vi "Get Thermocouple Meas Volt.vi"(8 "error in (no error)":errorcluster, 11 "VISA resource name":refnum<visa-resource-name>) -> (0 "error out":errorcluster, 2 "Meas Value":dbl format="%^.3e", 3 "VISA resource name out":refnum<visa-resource-name>)   [LabVIEW 2014, in "Fluke 5XXX Series Multicalibrators.lvlib"]
doc: "This VI returns the last value of the thermocouple temperature measurement in volts. If the last measurement was an overload or open thermocouple condition, or there is no measurement, returns 0E+00.\n\nNote:\n\nThis VI is available only for instrument models 5500A and 5520A."
uses:
  Fluke 5XXX Series Multicalibrators.lvlib
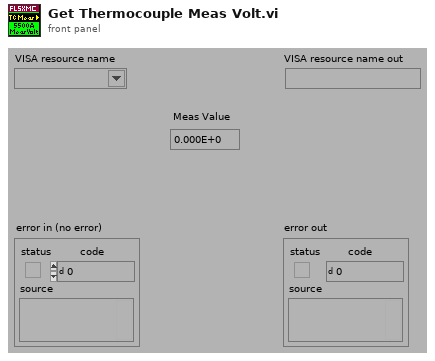
[diagram p1: front panel]
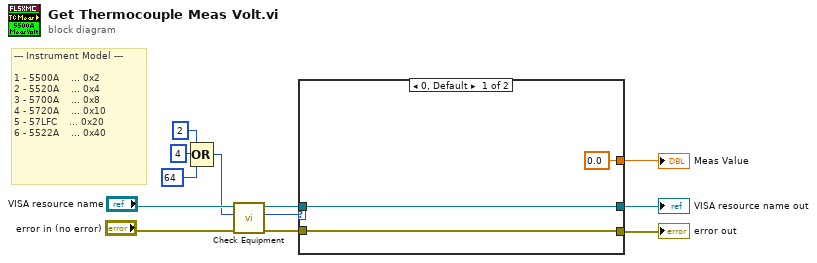
[diagram p0: block diagram]
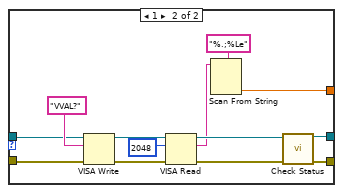
[diagram p2: hidden frame]
diagram:
  # "--- Instrument Model ---\n\n1 - 5500A    ... 0x2\n2 - 5520A    ... 0x4\n3 - 5700A    ... 0x8\n4 - 5720A    ... 0x10\n5 - 57LFC    ... 0x20\n6 - 5522A    ... 0x40"
  n1 = Compound Arithmetic op=OR(2 ("Numeric"), 4 ("Numeric"), 64 ("Numeric")) -> (w5:i32)
  n2 = call "Check Equipment.vi"("error in (no error)"="error in (no error)", "Bit Mask"=w5, "VISA resource name"="VISA resource name") -> ("error out"=w12:errorcluster, "Present?"=w10:u32, "VISA resource name out"=w11:refnum<visa-resource-name>)  [unwired: 6 in]
  n3 = case shown="0, Default" w10 {
    tunnel: [w15 w22] -> w3
    tunnel: [w14 w19] -> w2
    tunnel: w12 -> [w15 w24]
    tunnel: w11 -> [w14 w23]
    tunnel: [0.0 w16] -> w4
    frame 0, Default {
    }
    frame 1 {
      n4 = VISA Write(VISA resource name=w23, write buffer="VVAL?", error in (no error)=w24) -> (VISA resource name out=w27:refnum<visa-resource-name>, error out=w26:errorcluster)  [unwired: 1 out]
      n5 = VISA Read(VISA resource name=w27, byte count=u32 2048 ("byte count (0)"), error in (no error)=w26) -> (VISA resource name out=w20:refnum<visa-resource-name>, read buffer=w17:string, error out=w21:errorcluster)  [unwired: 1 out]
      n6 = Scan From String(format string="%.;%Le", input string=w17) -> (output 1=w16:dbl)  [unwired: 3 in, 3 out]
      n7 = call "Check Status.vi"("VISA resource name"=w20, "error in (no error)"=w21) -> ("VISA resource name out"=w19:refnum<visa-resource-name>, "error out"=w22:errorcluster)  [unwired: 12 in]
    }
  }
  "Meas Value" <- w4
  "VISA resource name out" <- w2
  "error out" <- w3
